vi "GSP_Manager_COLL_driver.vi"(4 "error in (no error)":errorcluster, 5 "Target (Move Only)":i32, 6 "Action":T1) -> (0 "error out":errorcluster, 3 "reference out (launch only)":refnum<vi>)   [LabVIEW 2015]
doc: "Provides an interface to the Collimator Focus Manager. See the actions below.\n\nLaunch - launch the manager thread supplying references to the controls that the thread will update.\n\nHome - Home the collimator focus manager\n\nMove - Move the collimator focus to the position supplied by Target\n\nShutdown - Shutdown the collimator focus manager"
uses:
  coll_actions.ctl
  SystemUtil/Command.ctl
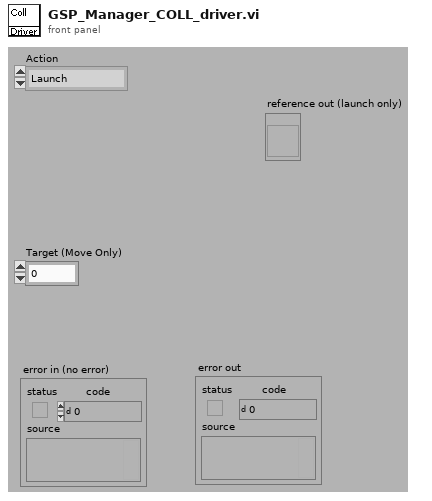
[diagram p1: front panel]
types:
  T1 = typedef "coll_actions.ctl" = enum16{"Launch", "Move", "Home", "Open Shutter", "Close Shutter", "Shutdown"}
  T2 = typedef "Command.ctl" = cluster{"Command":string, "Parameter":string}
  T3 = cluster{string, "type string":i16[], "data string":string}
  T4 = cluster{string, "type string":i16[], "data string":string}[]
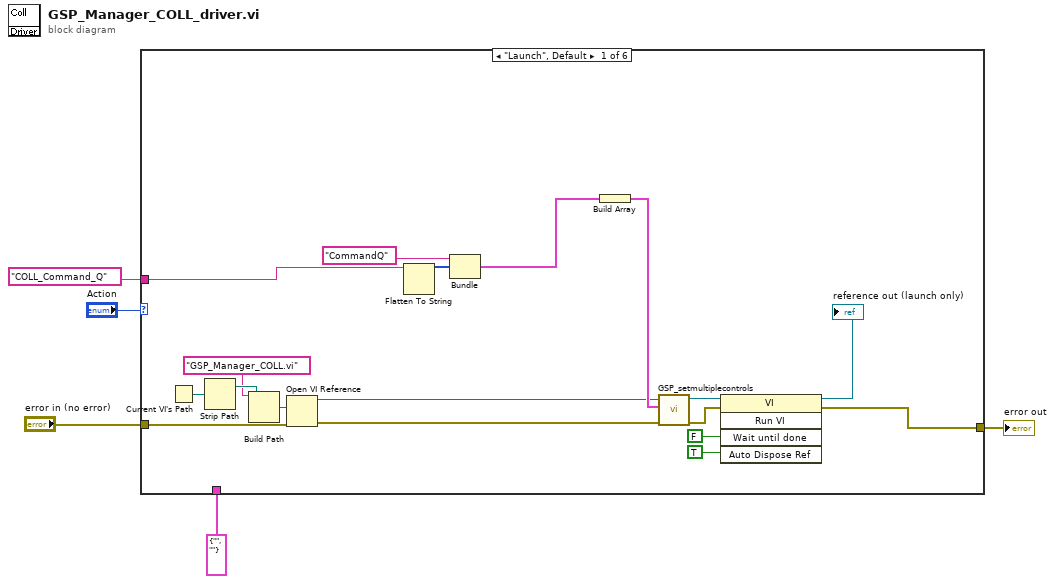
[diagram p0: block diagram]
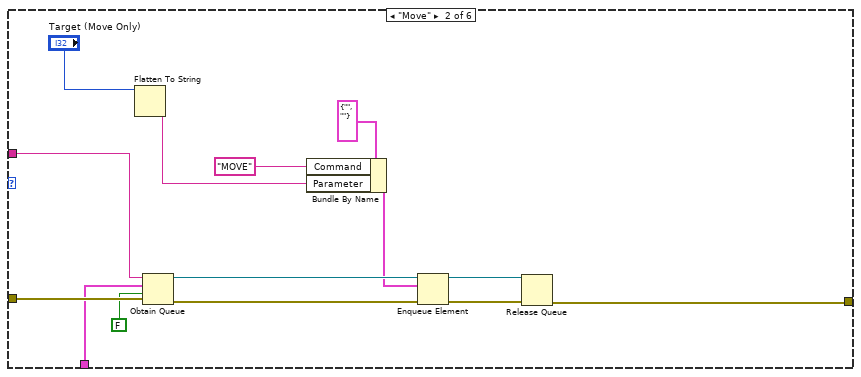
[diagram p2: hidden frame]
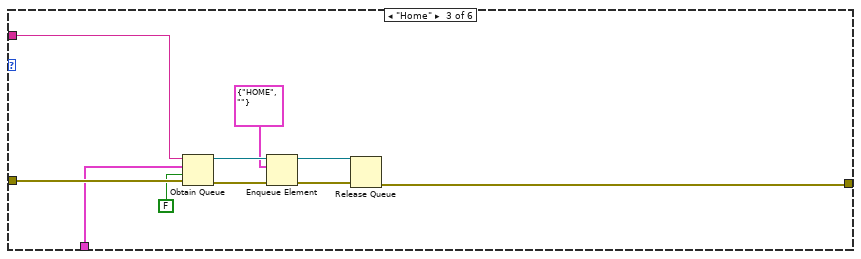
[diagram p3: hidden frame]
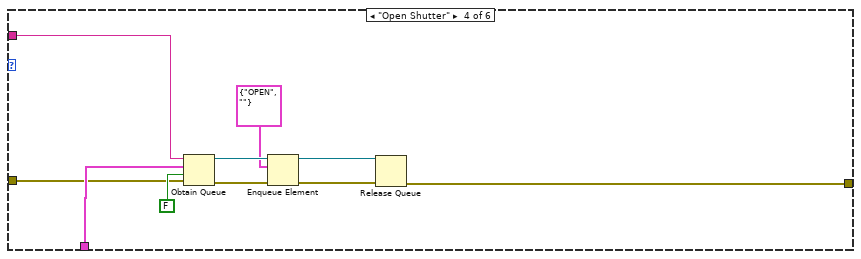
[diagram p4: hidden frame]
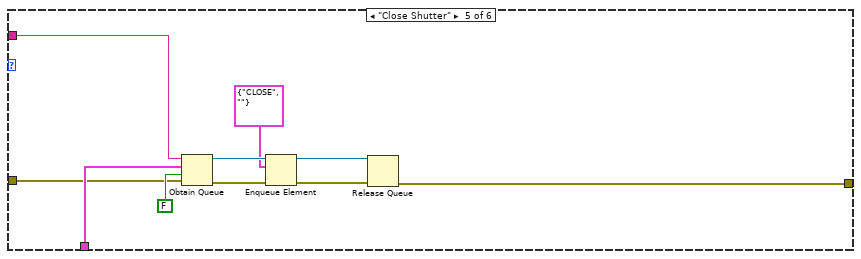
[diagram p5: hidden frame]
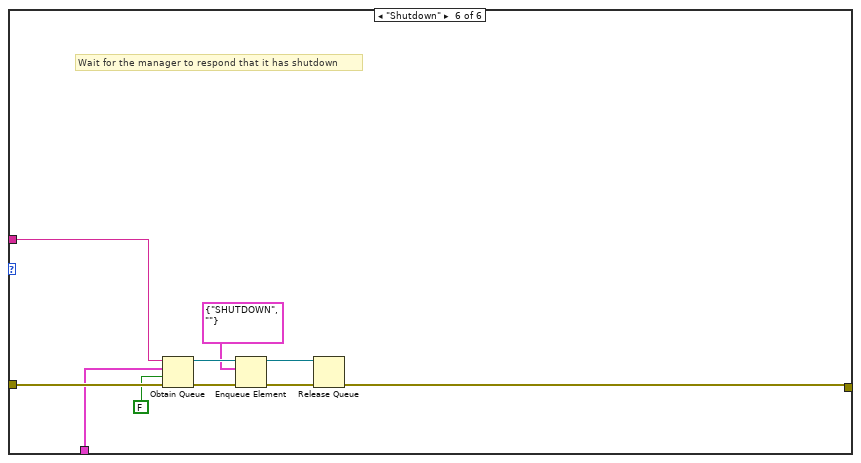
[diagram p6: hidden frame]
diagram:
  n1 = case shown="\"Launch\", Default" "Action" {
    tunnel: "error in (no error)" -> [w20 w38 w46 w53 w63 w78]
    tunnel: [w9 w25 w39 w49 w59 w69] -> w3
    tunnel: "COLL_Command_Q" -> [w10 w36 w45 w52 w62 w75]
    tunnel: T2 {"Command"="", "Parameter"=""} ("Command") -> [_ w33 w43 w54 w64 w73]
    frame "Launch", Default {
      n2 = Current VI's Path() -> (path=w14:path)
      n3 = Strip Path(path=w14) -> (stripped path=w12:path)  [unwired: 1 out]
      n4 = Build Path(base path=w12, name or relative path="GSP_Manager_COLL.vi" ("vi path")) -> (appended path=w13:path)
      n5 = Open VI Reference(vi path=w13, error in (no error)=w20) -> (vi reference=w8:refnum<vi>, error out=w19:errorcluster)  [unwired: 4 in]
      n6 = Flatten To String(anything=w10) -> (data string=w22:string, type string=w23:i16[])  [unwired: 3 in, 1 out]
      n7 = Bundle("CommandQ", "type string"=w23, "data string"=w22) -> (w7:T3)  [unwired: 1 in]
      n8 = Build Array(w7) -> (w21:T4)
      n9 = call "GSP_setmultiplecontrols.vi"("error in (no error)"=w19, "Control Infos"=w21, "reference"=w8) -> ("error out"=w17:errorcluster, "reference out"=w18:refnum<vi>)  [unwired: 3 in]
      n10 = invoke class="VI" method="Run VI"(reference=w18, error in=w17, "Wait until done"=FALSE, "Auto Dispose Ref"=TRUE) -> (reference out=→"reference out (launch only)":refnum<vi>, error out=w9:errorcluster)  [unwired: 1 in, 3 out]
    }
    frame "Move" {
      n11 = Flatten To String(anything="Target (Move Only)") -> (data string=w28:string)  [unwired: 3 in, 2 out]
      n12 = Obtain Queue(name (unnamed)=w36, element data type=w33, create if not found? (T)=FALSE, error in (no error)=w38) -> (queue out=w35:refnum<queue>, error out=w37:errorcluster)  [unwired: 1 in, 1 out]
      n13 = Bundle By Name(cluster=T2 {"Command"="", "Parameter"=""} ("element"), "Command"="MOVE" ("element"), "Parameter"=w28) -> (w31:T2)
      n14 = Enqueue Element(queue=w35, element=w31, error in (no error)=w37) -> (queue out=w27:refnum<queue>, error out=w26:errorcluster)  [unwired: 1 in, 1 out]
      n15 = Release Queue(queue=w27, error in (no error)=w26) -> (error out=w25:errorcluster)  [unwired: 1 in, 2 out]
    }
    frame "Home" {
      n16 = Obtain Queue(name (unnamed)=w45, element data type=w43, create if not found? (T)=FALSE, error in (no error)=w46) -> (queue out=w47:refnum<queue>, error out=w48:errorcluster)  [unwired: 1 in, 1 out]
      n17 = Enqueue Element(queue=w47, element=T2 {"Command"="HOME", "Parameter"=""}, error in (no error)=w48) -> (queue out=w41:refnum<queue>, error out=w40:errorcluster)  [unwired: 1 in, 1 out]
      n18 = Release Queue(queue=w41, error in (no error)=w40) -> (error out=w39:errorcluster)  [unwired: 1 in, 2 out]
    }
    frame "Open Shutter" {
      n19 = Obtain Queue(name (unnamed)=w52, element data type=w54, create if not found? (T)=FALSE, error in (no error)=w53) -> (queue out=w57:refnum<queue>, error out=w58:errorcluster)  [unwired: 1 in, 1 out]
      n20 = Enqueue Element(queue=w57, element=T2 {"Command"="OPEN", "Parameter"=""}, error in (no error)=w58) -> (queue out=w51:refnum<queue>, error out=w50:errorcluster)  [unwired: 1 in, 1 out]
      n21 = Release Queue(queue=w51, error in (no error)=w50) -> (error out=w49:errorcluster)  [unwired: 1 in, 2 out]
    }
    frame "Close Shutter" {
      n22 = Obtain Queue(name (unnamed)=w62, element data type=w64, create if not found? (T)=FALSE, error in (no error)=w63) -> (queue out=w67:refnum<queue>, error out=w68:errorcluster)  [unwired: 1 in, 1 out]
      n23 = Enqueue Element(queue=w67, element=T2 {"Command"="CLOSE", "Parameter"=""}, error in (no error)=w68) -> (queue out=w61:refnum<queue>, error out=w60:errorcluster)  [unwired: 1 in, 1 out]
      n24 = Release Queue(queue=w61, error in (no error)=w60) -> (error out=w59:errorcluster)  [unwired: 1 in, 2 out]
    }
    frame "Shutdown" {
      # "Wait for the manager to respond that it has shutdown"
      n25 = Obtain Queue(name (unnamed)=w75, element data type=w73, create if not found? (T)=FALSE, error in (no error)=w78) -> (queue out=w76:refnum<queue>, error out=w77:errorcluster)  [unwired: 1 in, 1 out]
      n26 = Enqueue Element(queue=w76, element=T2 {"Command"="SHUTDOWN", "Parameter"=""}, error in (no error)=w77) -> (queue out=w71:refnum<queue>, error out=w70:errorcluster)  [unwired: 1 in, 1 out]
      n27 = Release Queue(queue=w71, error in (no error)=w70) -> (error out=w69:errorcluster)  [unwired: 1 in, 2 out]
    }
  }
  "error out" <- w3
